vi "Get Local Destination Directory.vi"(8 "error in":errorcluster, 11 "Build Spec in":T1) -> (0 "error out":errorcluster, 3 "Build Spec out":T1, 4 "Local Destination Directory":path)   [LabVIEW 2019, in "Project Sync Tools.lvclass"]
uses:
  Project Sync Tools.lvclass
  TypeDefs/BuildSpec Parameters.ctl
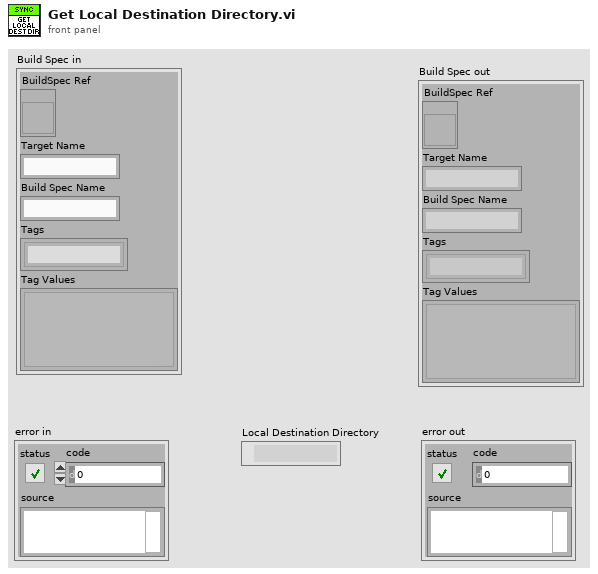
[diagram p1: front panel]
types:
  T1 = typedef "Project Sync Tools.lvclass/BuildSpec Parameters.ctl" = cluster{"BuildSpec Ref":refnum<vi>, "Target Name":string, "Build Spec Name":string, "Tags":string[], "Tag Values":variant[]}
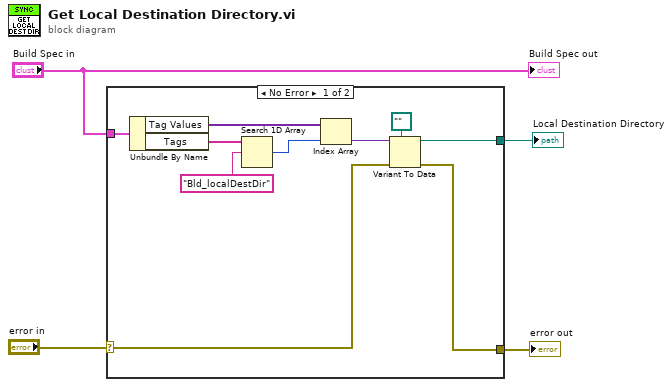
[diagram p0: block diagram]
diagram:
  n1 = case shown="No Error" "error in" {
    selector: "error in" -> [w5 w15]
    tunnel: "Build Spec in" -> [w10 _]
    tunnel: [w7 _] -> w3
    tunnel: [w6 w15] -> w2
    frame No Error {
      n2 = Unbundle By Name(w10) -> ("Tag Values"=w13:variant[], "Tags"=w11:string[])
      n3 = Search 1D Array(1D array=w11, element="Bld_localDestDir") -> (index of element=w14:i32)  [unwired: 1 in]
      n4 = Index Array(array=w13, index=w14) -> (element=w9:variant)
      n5 = Variant To Data(error in=w5, type=path "", Variant=w9) -> (data=w7:path, error out=w6:errorcluster)
    }
    frame Error {
    }
  }
  "Local Destination Directory" <- w3
  "error out" <- w2
  "Build Spec out" <- "Build Spec in"
